vi "搜索串口.vi"() -> ()   [LabVIEW 2015]
uses:
  <vilib>/Instr/_visa.llb/VISA Find Search Mode.ctl
panel:
  out "查找列表":string[](array[string])
  out "串口":cluster{string, string}[](array[cluster])
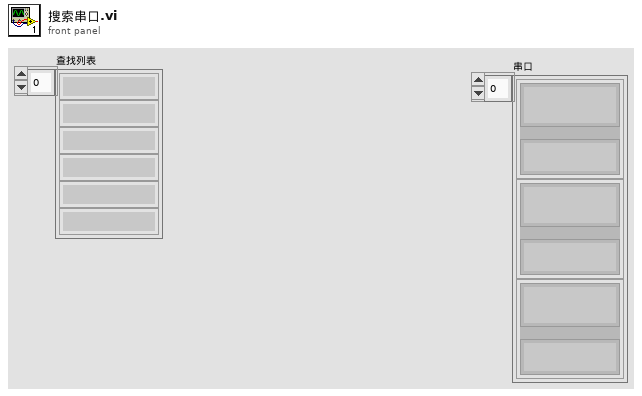
[diagram p1: front panel]
types:
  T1 = typedef "VISA Find Search Mode.ctl" = u32
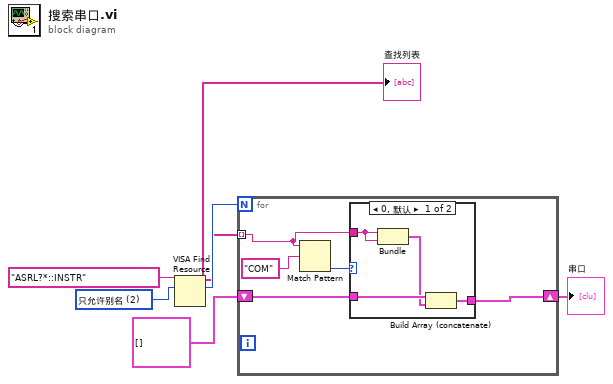
[diagram p0: block diagram]
diagram:
  w3 = T1 2 items=["仅允许规范名称"=0, "只允许别名"=2, "包含匹配别名"=3, "包含所有别名"=4] ("Search Mode")
  n1 = VISA Find Resource(10:w3, 11:"ASRL?*::INSTR") -> (2:w5:u32, 3:w4:string[])  [unwired: 1 in, 1 out]
  "查找列表" <- w4
  n2 = for {
    N: w5 -> [_]
    tunnel: w4 -> [w9] mode=indexing
    shift-right: [w8] -> w1
    shift-left: cluster{string, string}[] [] -> [w7]
    n3 = Match Pattern(string=w9, regular expression="COM" ("正则表达式")) -> (offset past match=w10:i32)  [unwired: 1 in, 3 out]
    n4 = case shown="0, 默认" w10 {
      tunnel: w7 -> [w15 w16]
      tunnel: w9 -> [w13 _]
      tunnel: [w14 w16] -> w8
      frame 0, Default {
        n5 = Bundle(w13, w13) -> (w12:cluster{string, string})  [unwired: 1 in]
        n6 = Build Array (concatenate)(w15, w12) -> (w14:cluster{string, string}[])
      }
      frame -1 {
      }
    }
  }
  "串口" <- w1
